vi "DP-Plot Data.vi"(0 "XYGraph":refnum<vi>, 7 "vs Freq":bool, 11 "f2":dbl[](array[numeric]), 12 "1st row current freq":i32, 13 "Input Array (4xn)":dbl[][](array[numeric]) format="%.2f") -> ()   [LabVIEW 2020]
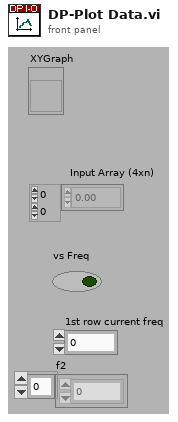
[diagram p1: front panel]
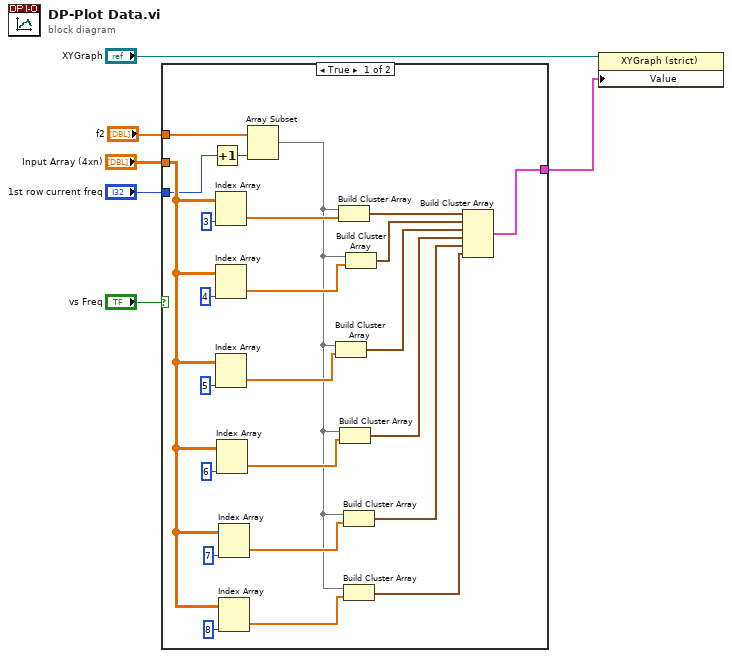
[diagram p0: block diagram]
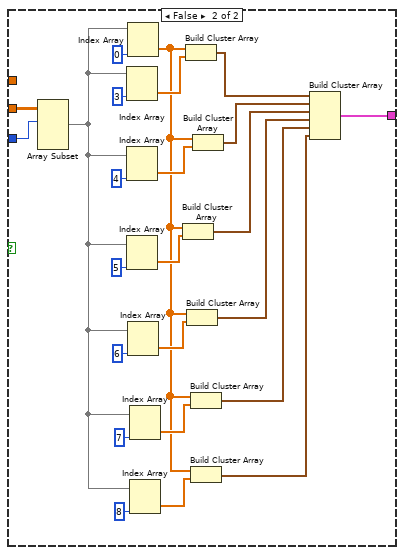
[diagram p2: hidden frame]
diagram:
  n1 = case shown="True" "vs Freq" {
    tunnel: "Input Array (4xn)" -> [w11 w33]
    tunnel: [w12 w34] -> w4
    tunnel: "1st row current freq" -> [w9 w32]
    tunnel: "f2" -> [w10 _]
    frame True {
      n2 = Increment(x=w9) -> (x+1=w7:i32)
      n3 = Index Array(array=w11, index (col)=3) -> (element=w28:dbl[])  [unwired: 1 in]
      n4 = Index Array(array=w11, index (col)=4) -> (element=w29:dbl[])  [unwired: 1 in]
      n5 = Index Array(array=w11, index (col)=5) -> (element=w23:dbl[])  [unwired: 1 in]
      n6 = Index Array(array=w11, index (col)=6) -> (element=w21:dbl[])  [unwired: 1 in]
      n7 = Index Array(array=w11, index (col)=7) -> (element=w17:dbl[])  [unwired: 1 in]
      n8 = Index Array(array=w11, index (col)=8) -> (element=w15:dbl[])  [unwired: 1 in]
      n9 = Array Subset(array=w10, length=w7) -> (w8:dbl[])  [unwired: 1 in]
      n10 = Build Cluster Array(w8, w23) -> (w22:cluster{"f2":dbl, dbl}[])
      n11 = Build Cluster Array(w8, w28) -> (w30:cluster{"f2":dbl, dbl}[])
      n12 = Build Cluster Array(w8, w21) -> (w19:cluster{"f2":dbl, dbl}[])
      n13 = Build Cluster Array(w8, w17) -> (w16:cluster{"f2":dbl, dbl}[])
      n14 = Build Cluster Array(w8, w15) -> (w13:cluster{"f2":dbl, dbl}[])
      n15 = Build Cluster Array(w8, w29) -> (w25:cluster{"f2":dbl, dbl}[])
      n16 = Build Cluster Array(w30, w25, w22, w19, w16, w13) -> (w12:cluster{cluster{"f2":dbl, dbl}[]}[])
    }
    frame False {
      n17 = Array Subset(array=w33, index (row)=w32) -> (w31:dbl[][])  [unwired: 3 in]
      n18 = Index Array(array=w31, index (col)=3) -> (element=w52:dbl[])  [unwired: 1 in]
      n19 = Index Array(array=w31, index (col)=4) -> (element=w53:dbl[])  [unwired: 1 in]
      n20 = Index Array(array=w31, index (col)=5) -> (element=w46:dbl[])  [unwired: 1 in]
      n21 = Index Array(array=w31, index (col)=0) -> (element=w36:dbl[])  [unwired: 1 in]
      n22 = Index Array(array=w31, index (col)=6) -> (element=w44:dbl[])  [unwired: 1 in]
      n23 = Index Array(array=w31, index (col)=7) -> (element=w40:dbl[])  [unwired: 1 in]
      n24 = Index Array(array=w31, index (col)=8) -> (element=w38:dbl[])  [unwired: 1 in]
      n25 = Build Cluster Array(w36, w46) -> (w45:cluster{dbl, dbl}[])
      n26 = Build Cluster Array(w36, w52) -> (w54:cluster{dbl, dbl}[])
      n27 = Build Cluster Array(w36, w44) -> (w42:cluster{dbl, dbl}[])
      n28 = Build Cluster Array(w36, w40) -> (w39:cluster{dbl, dbl}[])
      n29 = Build Cluster Array(w36, w38) -> (w35:cluster{dbl, dbl}[])
      n30 = Build Cluster Array(w36, w53) -> (w48:cluster{dbl, dbl}[])
      n31 = Build Cluster Array(w54, w48, w45, w42, w39, w35) -> (w34:cluster{cluster{dbl, dbl}[]}[])
    }
  }
  n32 = property class="XYGraph (strict)"(reference="XYGraph", "Value"=w4) -> ()  [unwired: 1 in, 2 out]
